vi "Clear_log.vi"(8 "error in (no error)":errorcluster, 11 "Actor_Log in":refnum<class "Actor_Log.lvclass">) -> (0 "error out":errorcluster, 3 "Actor_Log out":refnum<class "Actor_Log.lvclass">)   [LabVIEW 2020, in "Library Core.lvlib" / "Actor_Log.lvlib" / "Actor_Log.lvclass"]
uses:
  Actor_Log.lvclass
  Actor_Log.lvclass/Actor_Log.ctl
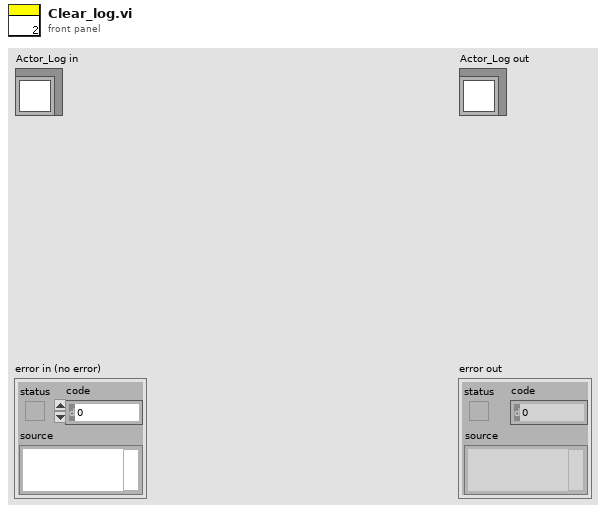
[diagram p1: front panel]
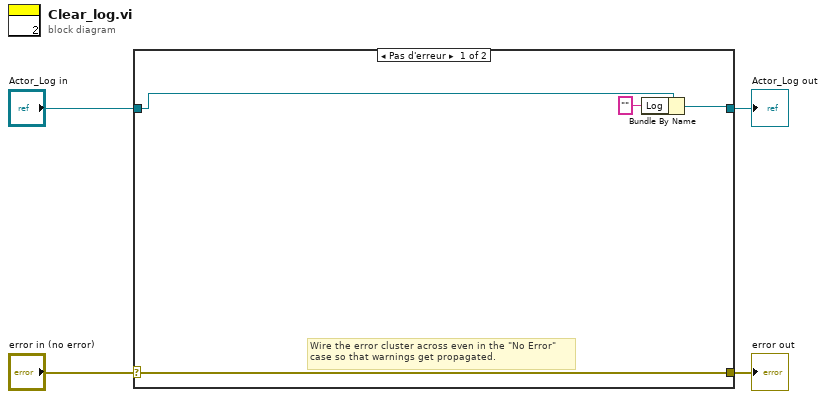
[diagram p0: block diagram]
diagram:
  n1 = case shown="Pas d'erreur" "error in (no error)" {
    selector: "error in (no error)" -> [w8 w10]
    tunnel: [w8 w10] -> w3
    tunnel: [w7 w9] -> w1
    tunnel: "Actor_Log in" -> [w6 w9]
    frame No Error {
      # "Wire the error cluster across even in the \"No Error\"\ncase so that warnings get propagated."
      n2 = Bundle By Name(cluster=w6, "Log"="") -> (w7:refnum<class "Actor_Log.lvclass">)
    }
    frame Error {
    }
  }
  "error out" <- w3
  "Actor_Log out" <- w1
